vi "TickTock.vi"(8 "Error In":errorcluster, 11 "Current Time (In)":timestamp) -> (0 "Error Out":errorcluster, 2 "dt":dbl, 3 "Current Time (Out)":timestamp)   [LabVIEW 2014]
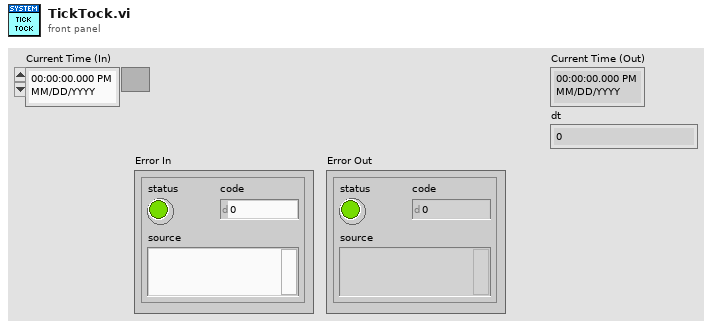
[diagram p1: front panel]
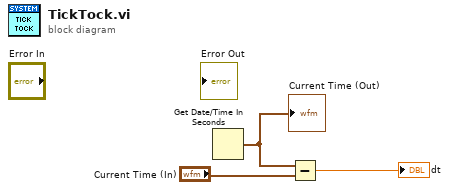
[diagram p0: block diagram]
diagram:
  n1 = Get Date/Time In Seconds() -> (seconds since 1Jan1904=w3:timestamp)
  "Current Time (Out)" <- w3
  n2 = Subtract(x=w3, y="Current Time (In)") -> (x-y=→"dt":dbl)
